vi "LanguageChanged.vi"(8 "error in":errorcluster, 10 "String":string, 11 "Module ID":i32=-1) -> (0 "error out":errorcluster)   [LabVIEW 2025, in "Test Unit.lvlib"]
doc: "_____\nCreated using DQMH Framework: Event Scripter 7.1.1.1528."
uses:
  Test Unit.lvlib
  LanguageChanged Argument--cluster.ctl
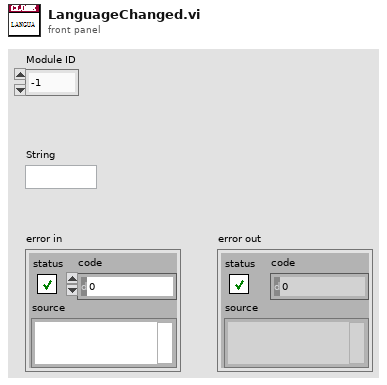
[diagram p1: front panel]
types:
  T1 = typedef "Test Unit.lvlib/LanguageChanged Argument--cluster.ctl" = cluster{"Module ID":i32, "String":string}
  T2 = typedef "Test Unit.lvlib/Request Events--cluster.ctl" = cluster{"Stop Module":refnum<user-event>, "Show Panel":refnum<user-event>, "Hide Panel":refnum<user-event>, "Show Diagram":refnum<user-event>, "Get Module Execution Status":refnum<user-event>, "TileWindows":refnum<user-event>, "TitleWindows":refnum<user-event>, "Cofiguration":refnum<user-event>, "Load Sequence":refnum<user-event>, "Write SN":refnum<user-event>, "UUT Test":refnum<user-event>, "UUTs Test":refnum<user-event>, "Terminate Test":refnum<user-event>, "Set Variable":refnum<user-event>, "Get Variable":refnum<user-event>, "LanguageChanged":refnum<user-event>}
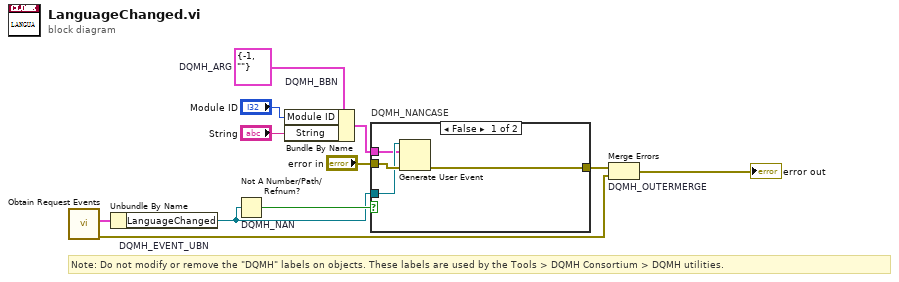
[diagram p0: block diagram]
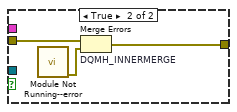
[diagram p2: hidden frame]
diagram:
  w5 = T1 {"Module ID"=-1, "String"=""}  # DQMH_ARG
  # "Note: Do not modify or remove the \"DQMH\" labels on objects. These labels are used by the Tools > DQMH Consortium > DQMH utilities."
  n1 = call "Obtain Request Events.vi"() -> ("error out"=w2:errorcluster, "Test Unit Request Events"=w1:T2)  [unwired: 10 in]
  n2 = Unbundle By Name "DQMH_EVENT_UBN"(w1) -> ("LanguageChanged"=w7:refnum<user-event>)
  n3 = Not A Number/Path/Refnum? "DQMH_NAN"(number/path/refnum=w7) -> (NaN/Path/Refnum?=w8:bool)
  n4 = Bundle By Name "DQMH_BBN"(cluster=w5, "Module ID"="Module ID", "String"="String") -> (w9:T1)
  n5 = case "DQMH_NANCASE" shown="False" w8 {
    tunnel: "error in" -> [w15 w18]
    tunnel: [w14 w17] -> w6
    tunnel: w7 -> [w13 _]
    tunnel: w9 -> [w12 _]
    frame False {
      n6 = Generate User Event(user event=w13, event data cluster=w12, error in=w15) -> (error out=w14:errorcluster)  [unwired: 1 in, 1 out]
    }
    frame True {
      n7 = call "Module Not Running--error.vi"() -> ("error out"=w16:errorcluster)  [unwired: 11 in]
      n8 = Merge Errors "DQMH_INNERMERGE"(w18, w16) -> (w17:errorcluster)
    }
  }
  n9 = Merge Errors "DQMH_OUTERMERGE"(w6, w2) -> (→"error out":errorcluster)
